vi "Get Class Methods from Object.vi"(0 "App Ref":refnum<vi>, 1 "object":refnum<class>, 3 "error in":errorcluster) -> (5 "Wire Pens":T1(array[cluster]), 6 "dup App Ref":refnum<vi>, 7 "Method Names":string[](array[string]), 8 "Method VIs":refnum<vi>[](array[refnum]), 9 "error out":errorcluster)   [LabVIEW 2025, in "XNode Support.lvlib"]
uses:
  XNode Support.lvlib
  <vilib>/regexp/Match Regular Expression.xnode
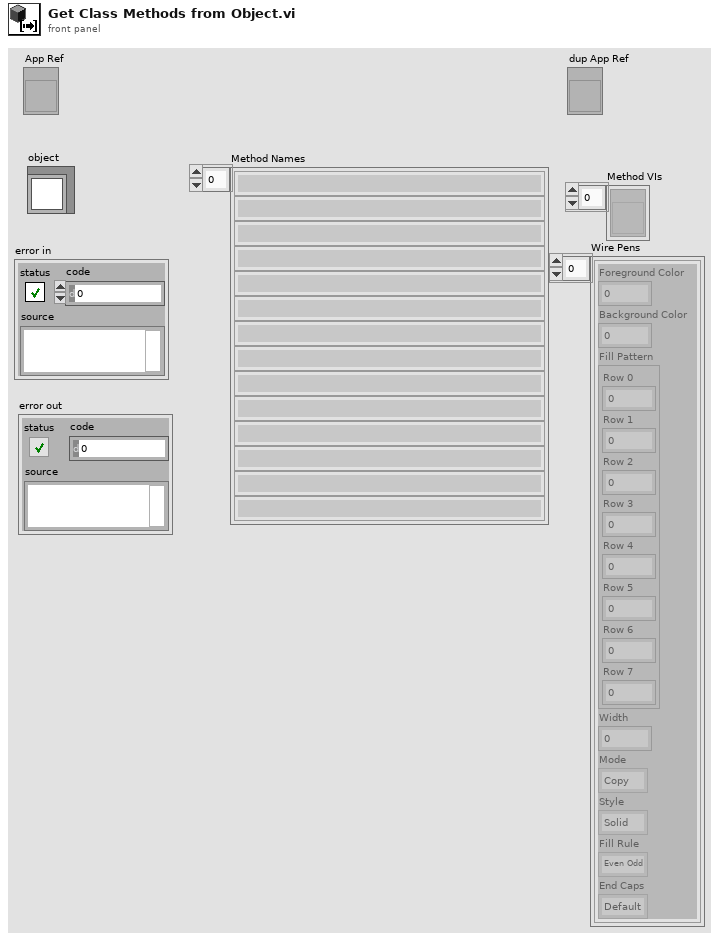
[diagram p1: front panel]
types:
  T1 = cluster{"Foreground Color":u32, "Background Color":u32, "Fill Pattern":cluster{"Row 0":u8, "Row 1":u8, "Row 2":u8, "Row 3":u8, "Row 4":u8, "Row 5":u8, "Row 6":u8, "Row 7":u8}, "Width":i16, "Mode":enum16{"Copy", "Or", "Exclusive Or", "Bit Clear", "Not Copy", "Not Or", "Nor Exclusive Or", "Not Bit Clear"}, "Style":enum32{"Solid", "Dash", "Dot", "Dash Dot", "Dash Dot Dot"}, "Fill Rule":enum32{"Even Odd", "Winding"}, "End Caps":enum32{"Default", "Flat"}}[]
  T2 = enum32{"invalid VI type", "Standard VI", "Control VI", "Global VI", "Polymorphic VI", "Configuration VI", "SubSystem", "Facade VI", "Method VI", "Statechart Diagram VI"}
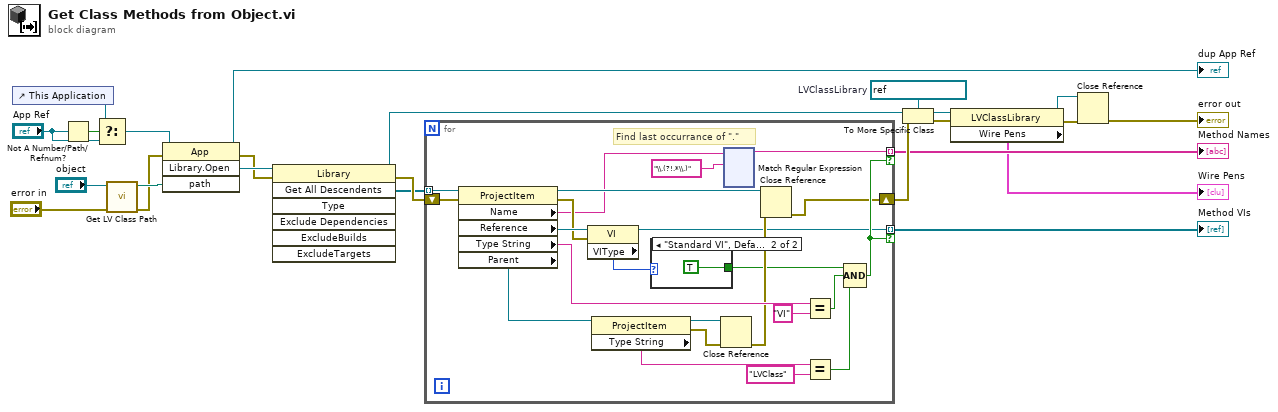
[diagram p0: block diagram]
diagram:
  w12 = refnum<vi> refnum  # LVClassLibrary
  n1 = control-ref of="This Application"() -> (w16:refnum<vi>)
  n2 = Not A Number/Path/Refnum?(number/path/refnum="App Ref") -> (NaN/Path/Refnum?=w17:bool)
  n3 = Select(t=w16, s=w17, f="App Ref") -> (s? t:f=w15:refnum<vi>)
  n4 = call <vilib>:"Get LV Class Path.vi"("error in (no error)"="error in", "object"="object") -> ("error out"=w23:errorcluster, "class path"=w24:path)  [unwired: 8 in]
  n5 = invoke class="App" method="Library.Open"(reference=w15, error in=w23, "path"=w24) -> (reference out=→"dup App Ref":refnum<vi>, error out=w20:errorcluster, "Open Library"=w22:refnum<vi>)  [unwired: 1 in, 1 out]
  n6 = invoke class="Library" method="Get All Descendents"(reference=w22, error in=w20) -> (reference out=w5:refnum<vi>, error out=w7:errorcluster, "All Descendents"=w6:refnum<vi>[])  [unwired: 5 in, 4 out]
  n7 = for {
    tunnel: w6 -> [w47] mode=indexing
    tunnel: [w31] -> w2 mode=indexing if=w39
    tunnel: [w25] -> w3 mode=indexing if=w39
    shift-right: [w33] -> w13
    shift-left: w7 -> [w38]
    # "Find last occurrance of \".\""
    n8 = property class="ProjectItem"(reference=w47, error in=w38) -> (reference out=w35:refnum<vi>, error out=w30:errorcluster, "Name"=w26:string, "Reference"=w32:refnum<vi>, "Type String"=w45:string, "Parent"=w46:refnum<vi>)
    n9 = property class="VI"(reference=w32, error in=w30) -> (reference out=w31:refnum<vi>, "VIType"=w29:T2)  [unwired: 1 out]
    n10 = property class="ProjectItem"(reference=w46) -> (reference out=w37:refnum<vi>, error out=w36:errorcluster, "Type String"=w44:string)  [unwired: 1 in]
    n11 = case shown="\"Standard VI\", Default" w29 {
      tunnel: [_ TRUE] -> w28
      frame "invalid VI type", "Control VI", "Global VI" {
      }
      frame "Standard VI", Default {
      }
    }
    n12 = Close Reference(reference=w37, error in (no error)=w36) -> (error out=w34:errorcluster)
    n13 = xnode "Match Regular Expression"("input string"=w26, "regular expression"="\\.(?!.*\\.)") -> ("before match"=w25:string)  [unwired: 4 in, 4 out]
    n14 = Close Reference(reference=w35, error in (no error)=w34) -> (error out=w33:errorcluster)
    n15 = Equal?(x=w45, y="VI") -> (x = y?=w41:bool)
    n16 = Equal?(x=w44, y="LVClass") -> (x = y?=w40:bool)
    n17 = Compound Arithmetic op=AND(w28, w41, w40) -> (w39:bool)
  }
  "Method Names" <- w3
  "Method VIs" <- w2
  n18 = To More Specific Class(target class=w12, reference=w5, error in=w13) -> (specific class reference=w11:refnum<vi>, error out=w10:errorcluster)
  n19 = property class="LVClassLibrary"(reference=w11, error in=w10) -> (reference out=w8:refnum<vi>, error out=w9:errorcluster, "Wire Pens"=→"Wire Pens":T1)
  n20 = Close Reference(reference=w8, error in (no error)=w9) -> (error out=→"error out":errorcluster)
